vi "CU_InitClassifier.vi"(6 "ClassifierType":T2=enum."SVM Committee", 7 "Classifier Metaparameter":dbl, 8 "error in (no error)":errorcluster, 9 "Kernel Options":T3={"Kernel"=enum."RBF", "Degree"=3, "Gamma"=1.0, "Coefficient"=0.0, "Sigma"=1.0, "Cache(MB)"=10.0}, 10 "Paths":T4={"Training Data"=path "C:/Users/Paradise/Documents/BCI_project/raw_data_emotiv/O3VR/training data/ShortTimeFourierTransform_13.11.13_11-52.xml", "Test Data"=path "C:/Users/Paradise/Documents/BCI_project/raw_data_emotiv/O3VR/test data/ShortTimeFourierTransform_13.11.13_11-52.xml", "Test True Labels"=path "C:/Users/Paradise/Documents/BCI_project/raw_data_emotiv/O3VR/test data/true_labels_O3VR.txt"}, 11 "ClassifierClass in":refnum<class "ClassifierClass.lvclass">) -> (0 "error out":errorcluster, 2 "Number of Trials":T1, 3 "ClassifierClass out":refnum<class "ClassifierClass.lvclass">)   [LabVIEW 2016, in "Classifier.lvlib" / "ClassifierClass.lvclass"]
uses:
  ClassifierClass.lvclass
  <vilib>/vision/Classification.llb/IMAQ SVM Kernel Options.ctl
  CU_ClassifierTypes.ctl
  ClassifierClass.lvclass/ClassifierClass.ctl
  <vilib>/Utility/file.llb/Read Delimited Spreadsheet (string).vi
  <vilib>/xml/Load XML File.vi
  <vilib>/xml/NI_XML.lvlib
  _XML_EEG_Features/XML_EEG_Features.lvlib
  Classifier.lvlib
panel:
  # "This VI is a part of BCI Design library, http://www.ru-bci.org \nCopyright © 2020, Sotnikov Peter, All rights reserved. License: GNU GPLv3"
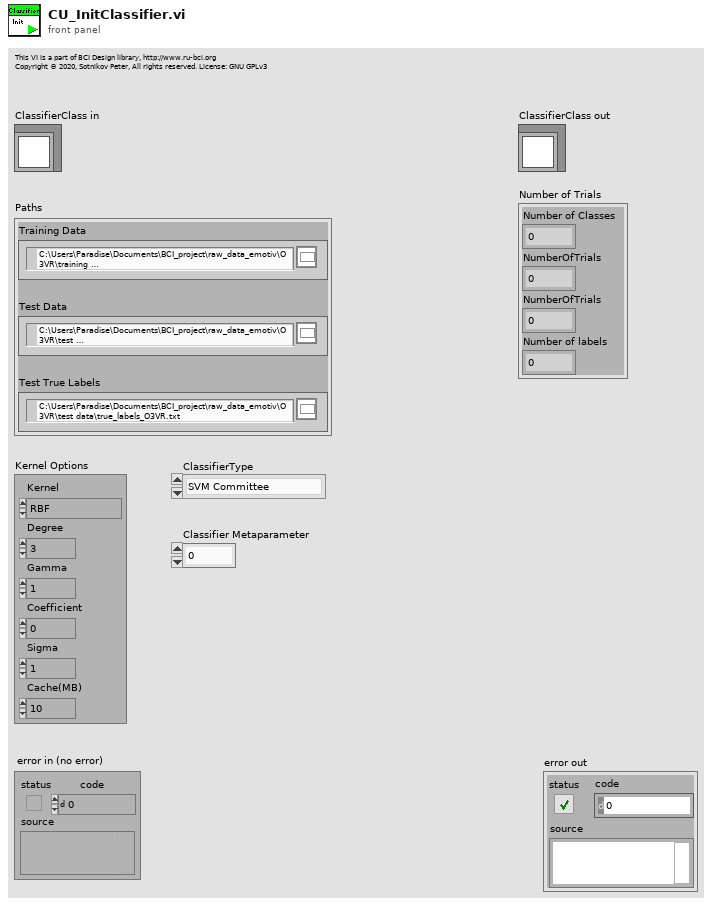
[diagram p1: front panel]
types:
  T1 = cluster{"Number of Classes":i32, "NumberOfTrials":i32, "NumberOfTrials":i32, "Number of labels":i32}
  T2 = typedef "Classifier.lvlib/CU_ClassifierTypes.ctl" = enum16{"Multilayer perceptron", "k NN Classifier", "SVM Committee", "Mahalanobis distance", "SVM Classifier"}
  T3 = typedef "IMAQ SVM Kernel Options.ctl" = cluster{"Kernel":enum32{"Linear", "Polynomial", "Gaussian", "RBF"}, "Degree":i32, "Gamma":dbl, "Coefficient":dbl, "Sigma":dbl, "Cache(MB)":dbl}
  T4 = cluster{"Training Data":path, "Test Data":path, "Test True Labels":path}
  T5 = typedef "XML_EEG_Features.lvlib/XML_FF_Header.ctl" = cluster{"NumberOfTrials":i32, "NumberOfClasses":i32, "FeatureVectorLength":i32, "FeatureExtractionMethod":string}
  T6 = cluster{i32, "NumberOfTrials":i32, "NumberOfTrials":i32, i32}
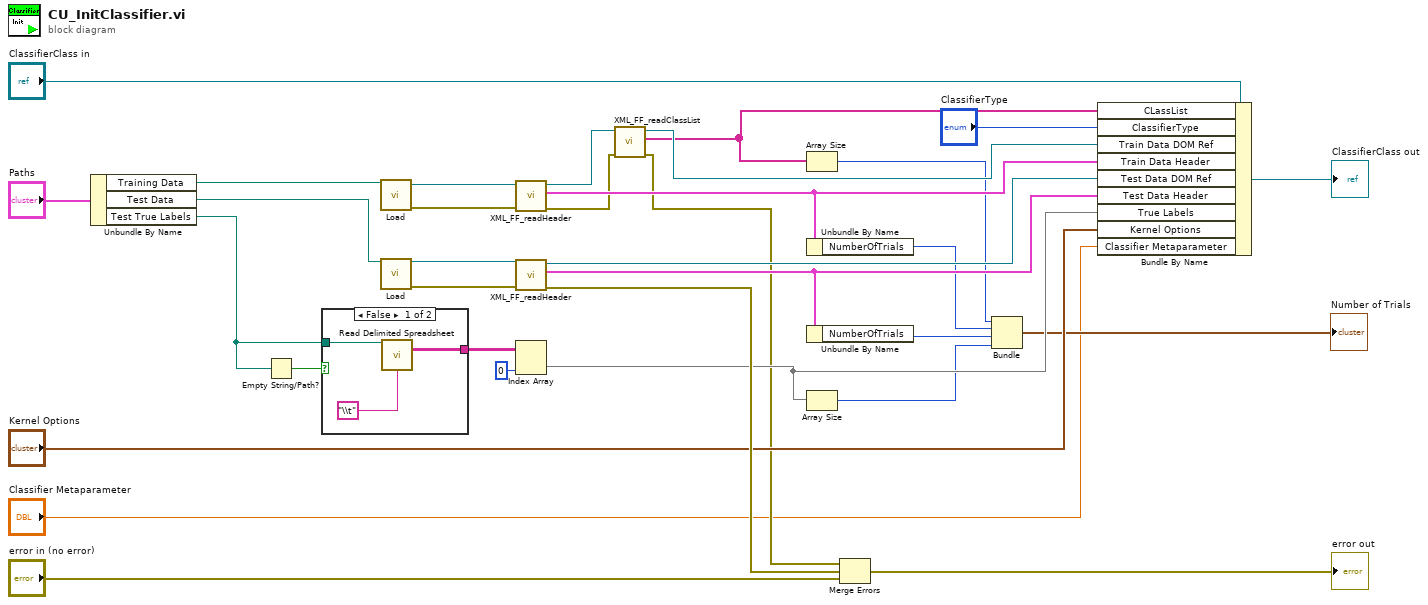
[diagram p0: block diagram]
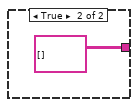
[diagram p2: hidden frame]
diagram:
  n1 = Unbundle By Name("Paths") -> ("Training Data"=w32:path, "Test Data"=w29:path, "Test True Labels"=w3:path)
  n2 = Empty String/Path?(string/path=w3) -> (empty?=w2:bool)
  n3 = case shown="False" w2 {
    tunnel: w3 -> [w36 _]
    tunnel: [w34 string[][] [] ("all rows")] -> w4
    frame False {
      n4 = call-poly <vilib>:"Read Delimited Spreadsheet.vi"("file path (dialog if empty)"=w36, "delimiter (\\t)"="\\t" ("delimiter (\\t)")) -> ("all rows"=w34:string[][])  [unwired: 8 in, 5 out]
    }
    frame True {
    }
  }
  n5 = call-poly <vilib>:"Load.vi"("path to XML document"=w32) -> ("DOM document out"=w31:refnum<k20>, "error out"=w30:errorcluster)  [unwired: 12 in, 1 out]
  n6 = call-poly <vilib>:"Load.vi"("path to XML document"=w29) -> ("DOM document out"=w28:refnum<k20>, "error out"=w27:errorcluster)  [unwired: 12 in, 1 out]
  n7 = call "XML_FF_readHeader.vi"("error in (no error)"=w30, "DOM document in"=w31) -> ("error out"=w9:errorcluster, "FF_Header out"=w19:T5, "DOM document out"=w11:refnum<k20>)  [unwired: 7 in]
  n8 = call "XML_FF_readHeader.vi"("error in (no error)"=w27, "DOM document in"=w28) -> ("error out"=w26:errorcluster, "FF_Header out"=w18:T5, "DOM document out"=w24:refnum<k20>)  [unwired: 7 in]
  n9 = Index Array(array=w4, index (col)=0 ("disabled index (col)")) -> (element=w17:string[])  [unwired: 1 in]
  n10 = call "XML_FF_readClassList.vi"("error in (no error)"=w9, "DOM document in"=w11) -> ("error out"=w8:errorcluster, "CLassLabels out"=w7:string[], "DOM document out"=w10:refnum<k20>)  [unwired: 7 in]
  n11 = Array Size(array=w7) -> (size(s)=w6:i32)
  n12 = Unbundle By Name(w19) -> ("NumberOfTrials"=w16:i32)
  n13 = Unbundle By Name(w18) -> ("NumberOfTrials"=w15:i32)
  n14 = Array Size(array=w17) -> (size(s)=w14:i32)
  n15 = Merge Errors(w8, w26, "error in (no error)") -> (→"error out":errorcluster)
  n16 = Bundle(w6, "NumberOfTrials"=w16, "NumberOfTrials"=w15, w14) -> (→"Number of Trials":T6)  [unwired: 1 in]
  n17 = Bundle By Name(cluster="ClassifierClass in", "CLassList"=w7, "ClassifierType"="ClassifierType", "Train Data DOM Ref"=w10, "Train Data Header"=w19, "Test Data DOM Ref"=w24, "Test Data Header"=w18, "True Labels"=w17, "Kernel Options"="Kernel Options", "Classifier Metaparameter"="Classifier Metaparameter") -> (→"ClassifierClass out":refnum<class "ClassifierClass.lvclass">)
